vi "mxwScript_API_XMLTemplateName_DropBelowPreviousTemplate.vi"(8 "error in (no error)":errorcluster, 10 "distance":i32 min=0, 11 "absolutePath":string) -> (0 "error out":errorcluster, 3 "encoded absolutePath":string)   [LabVIEW 2020]
doc: "Add diagram to drop this template into to the template name."
uses:
  codeGenAPISupport.llb/cgAPI_mxwScript_DrpTmplt_SimpleDirection.ctl
  codeGenAPISupport.llb/cgAPI_mxwScript_DrpTmplt_TargetRefType.ctl
  codeGenAPISupport.llb/cgAPI_mxwScript_DrpTmplt_TargetRefTemplateData.ctl
  codeGenAPISupport.llb/cgAPI_mxwScript_DrpTmplt_TargetRefTemplateType.ctl
  codeGenAPISupport.llb/cgAPI_mxwScript_DrpTmplt_ReferencePosition.ctl
  codeGenAPISupport.llb/cgAPI_mxwScript_DrpTmplt_TerminalData.ctl
  codeGenAPISupport.llb/cgAPI_mxwScript_DrpTmplt_TemplateRefType.ctl
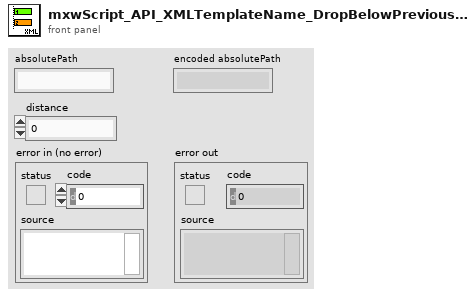
[diagram p1: front panel]
types:
  T1 = typedef "cgAPI_mxwScript_DrpTmplt_ReferencePosition.ctl" = enum16{"TopLeft", "Top", "TopRight", "Left", "Middle", "Right", "BottomLeft", "Bottom", "BottomRight"}
  T2 = typedef "cgAPI_mxwScript_DrpTmplt_TemplateRefType.ctl" = enum16{"InputAverage", "Absolute", "Terminal"}
  T3 = typedef "cgAPI_mxwScript_DrpTmplt_TargetRefTemplateType.ctl" = enum16{"OutputAverage", "Absolute", "Terminal"}
  T4 = typedef "cgAPI_mxwScript_DrpTmplt_TargetRefTemplateData.ctl" = cluster{"tag":string, "index":i32, "targetRefTemplateType":T3, "referencePosition":T1, "terminalData":T5}
  T5 = typedef "cgAPI_mxwScript_DrpTmplt_TerminalData.ctl" = cluster{"name":string, "termIsTag":bool, "referencePosition":T1}
  T6 = typedef "cgAPI_mxwScript_DrpTmplt_TargetRefType.ctl" = enum16{"RelativeToTemplate", "RelativeToTerminal", "AbsoluteOnRoot", "AbsoluteOnTarget", "RelativeToExistOnRoot"}
  T7 = typedef "cgAPI_mxwScript_DrpTmplt_SimpleDirection.ctl" = enum16{"Right", "Left", "Below", "Above"}
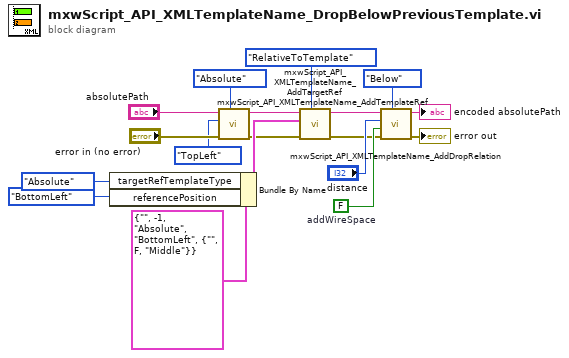
[diagram p0: block diagram]
diagram:
  w14 = FALSE  # addWireSpace
  n1 = Bundle By Name(cluster=T4 {"tag"="", "index"=-1, "targetRefTemplateType"=enum."Absolute", "referencePosition"=enum."BottomLeft", "terminalData"={"name"="", "termIsTag"=FALSE, "referencePosition"=enum."Middle"}} ("templateData"), "targetRefTemplateType"=cgAPI_mxwScript_DrpTmplt_TargetRefTemplateType."Absolute", "referencePosition"=cgAPI_mxwScript_DrpTmplt_ReferencePosition."BottomLeft") -> (w9:T4)
  n2 = call "mxwScript_API_XMLTemplateName_AddTemplateRef.vi"("templateRefType"=cgAPI_mxwScript_DrpTmplt_TemplateRefType."Absolute", "error in (no error)"="error in (no error)", "referencePosition"=cgAPI_mxwScript_DrpTmplt_ReferencePosition."TopLeft", "absolutePath"="absolutePath") -> ("error out"=w6:errorcluster, "encoded absolutePath"=w5:string)  [unwired: 1 in, 5 out]
  n3 = call "mxwScript_API_XMLTemplateName_AddTargetRef.vi"("targetRefType"=cgAPI_mxwScript_DrpTmplt_TargetRefType."RelativeToTemplate", "error in (no error)"=w6, "templateData"=w9, "absolutePath"=w5) -> ("error out"=w13:errorcluster, "encoded absolutePath"=w12:string)  [unwired: 3 in, 3 out]
  n4 = call "mxwScript_API_XMLTemplateName_AddDropRelation.vi"("direction"=cgAPI_mxwScript_DrpTmplt_SimpleDirection."Below", "error in (no error)"=w13, "addWireSpace"=w14, "distance"="distance", "absolutePath"=w12) -> ("error out"=→"error out":errorcluster, "encoded absolutePath"=→"encoded absolutePath":string)  [unwired: 5 out]
